vi "test_SimulatedScope SimulatedFGen on MSS ref in parallel.vi"(8 "Error In":errorcluster) -> (0 "Error Out":errorcluster)   [LabVIEW 2023]
uses:
  Measure and Stimulus Subsystems/Measure and Stimulus Subsystems.lvclass
panel:
  out "Photosensor Waveform Chart":waveform(dbl)(graph)
  in  "Stop":bool
  out "Powersensor Scalar":dbl
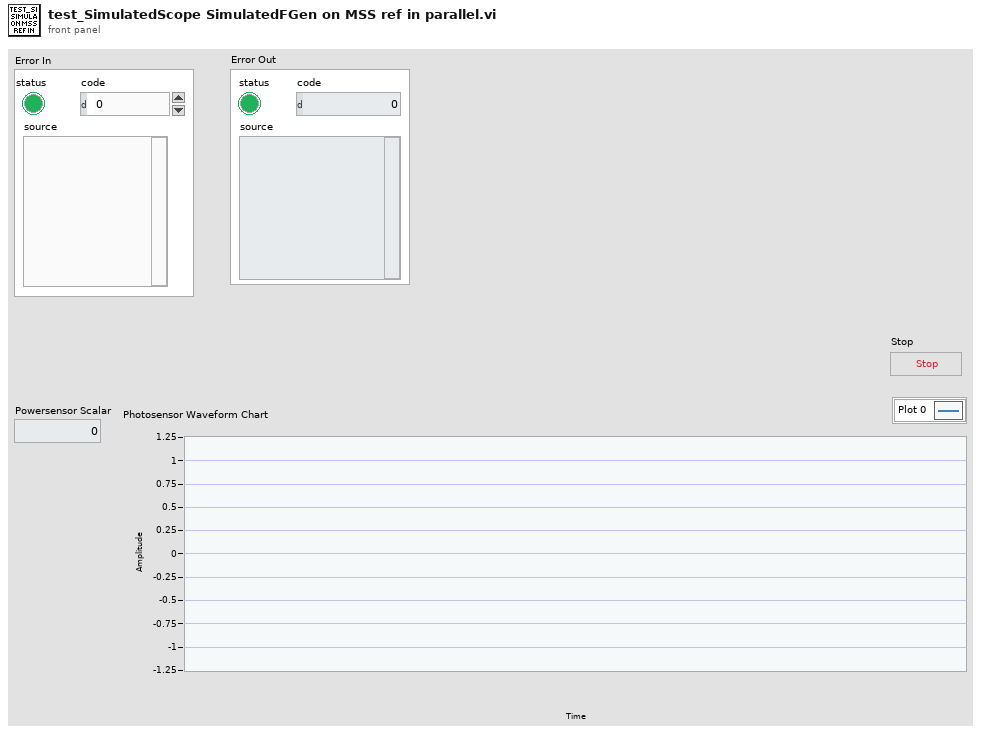
[diagram p1: front panel]
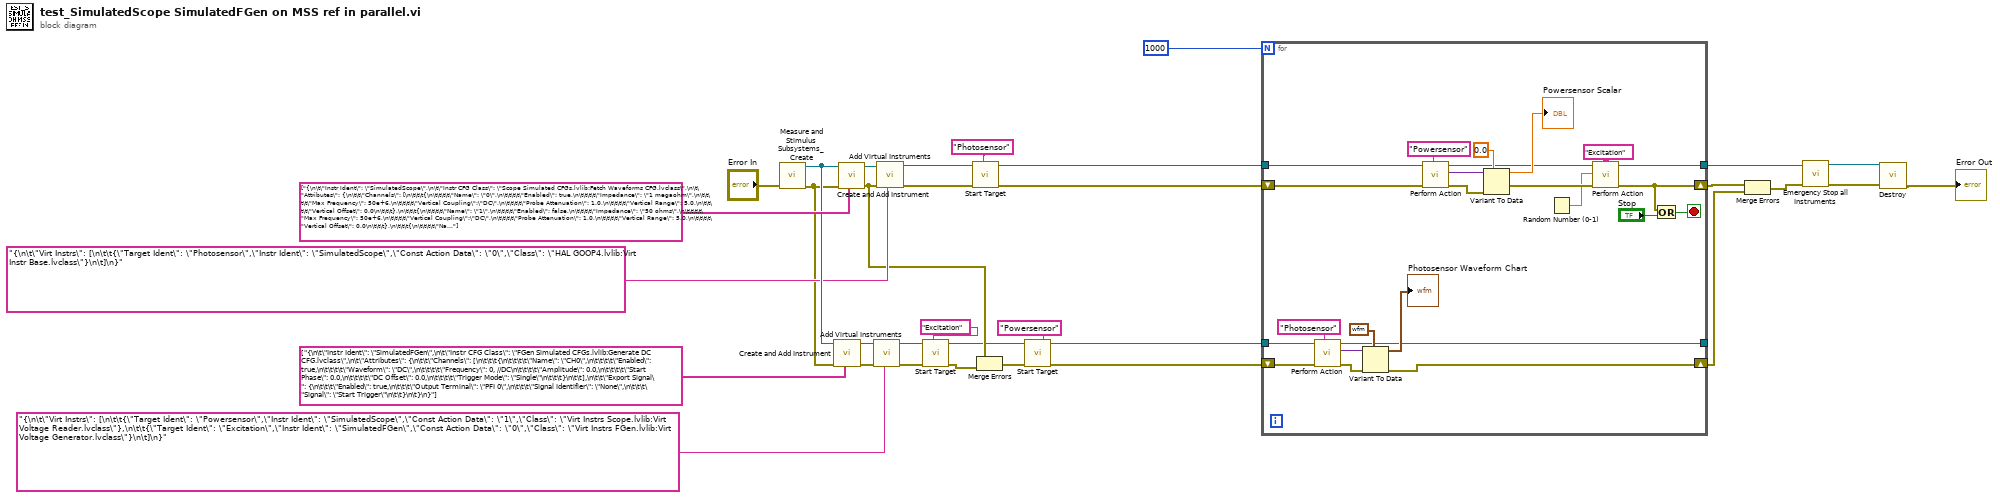
[diagram p0: block diagram]
diagram:
  n1 = call "Measure and Stimulus Subsystems_Create.vi"("Error In"="Error In") -> ("Error Out"=w16:errorcluster, "reference out"=w22:refnum<class "Measure and Stimulus Subsystems.lvclass">)  [unwired: 9 in]
  n2 = call "Create and Add Instrument.vi"("Physical Intr Configs"=string[] ["{\n\t\"Instr Ident\": \"SimulatedFGen\",\n\t\"Instr CFG Class\": \"FGen Simulated CFGs.lvlib:Generate DC CFG.lvclass\",\n\t\"Attributes\": {\n\t\t\"Channels\": [\n\t\t\t{\n\t\t\t\t\"Name\": \"CH0\",\n\t\t\t\t\"Enabled\": true,\n\t\t\t\t\"Waveform\": \"DC\",\n\t\t\t\t\"Frequency\": 0, //DC\n\t\t\t\t\"Amplitude\": 0.0,\n\t\t\t\t\"Start Phase\": 0.0,\n\t\t\t\t\"DC Offset\": 0.0,\n\t\t\t\t\"Trigger Mode\": \"Single\"\n\t\t\t}\n\t\t],\n\t\t\"Export Signal\": {\n\t\t\t\"Enabled\": true,\n\t\t\t\"Output Terminal\": \"PFI 0\",\n\t\t\t\"Signal Identifier\": \"None\",\n\t\t\t\"Signal\": \"Start Trigger\"\n\t\t}\n\t}\n}"], "Error In"=w16, "reference in"=w22) -> ("Error Out"=w15:errorcluster, "reference out"=w14:refnum<class "Measure and Stimulus Subsystems.lvclass">)  [unwired: 7 in]
  n3 = call "Create and Add Instrument.vi"("Physical Intr Configs"=string[] ["{\n\t\"Instr Ident\": \"SimulatedScope\",\n\t\"Instr CFG Class\": \"Scope Simulated CFGs.lvlib:Fetch Waveforms CFG.lvclass\",\n\t\"Attributes\": {\n\t\t\"Channels\": [\n\t\t\t{\n\t\t\t\t\"Name\": \"0\",\n\t\t\t\t\"Enabled\": true,\n\t\t\t\t\"Impedance\": \"1 megaohm\",\n\t\t\t\t\"Max Frequency\": 50e+6,\n\t\t\t\t\"Vertical Coupling\":\"DC\",\n\t\t\t\t\"Probe Attenuation\": 1.0,\n\t\t\t\t\"Vertical Range\": 5.0,\n\t\t\t\t\"Vertical Offset\": 0.0\n\t\t\t},\n\t\t\t{\n\t\t\t\t\"Name\": \"1\",\n\t\t\t\t\"Enabled\": false,\n\t\t\t\t\"Impedance\": \"50 ohms\",\n\t\t\t\t\"Max Frequency\": 50e+6,\n\t\t\t\t\"Vertical Coupling\":\"DC\",\n\t\t\t\t\"Probe Attenuation\": 1.0,\n\t\t\t\t\"Vertical Range\": 5.0,\n\t\t\t\t\"Vertical Offset\": 0.0\n\t\t\t},\n\t\t\t{\n\t\t\t\t\"Name\": \"2\",\n\t\t\t\t\"Enabled\": false,\n\t\t\t\t\"Impedance\": \"50 ohms\",\n\t\t\t\t\"Max Frequency\": 50e+6,\n\t\t\t\t\"Vertical Coupling\":\"DC\",\n\t\t\t\t\"Probe Attenuation\": 1.0,\n\t\t\t\t\"Vertical Range\": 5.0,\n\t\t\t\t\"Vertical Offset\": 0.0\n\t\t\t},\n\t\t\t{\n\t\t\t\t\"Name\": \"3\",\n\t\t\t\t\"Enabled\": true,\n\t\t\t\t\"Impedance\": \"50 ohms\",\n\t\t\t\t\"Max Frequency\": 50e+6,\n\t\t\t\t\"Vertical Coupling\":\"DC\",\n\t\t\t\t\"Probe Attenuation\": 1.0,\n\t\t\t\t\"Vertical Range\": 1.4,\n\t\t\t\t\"Vertical Offset\": 0.0\n\t\t\t},\n\t\t\t{\n\t\t\t\t\"Name\": \"4\",\n\t\t\t\t\"Enabled\": false,\n\t\t\t\t\"Impedance\": \"50 ohms\",\n\t\t\t\t\"Max Frequency\": 50e+6,\n\t\t\t\t\"Vertical Coupling\":\"DC\",\n\t\t\t\t\"Probe Attenuation\": 1.0,\n\t\t\t\t\"Vertical Range\": 5.0,\n\t\t\t\t\"Vertical Offset\": 0.0\n\t\t\t},\n\t\t\t{\n\t\t\t\t\"Name\": \"5\",\n\t\t\t\t\"Enabled\": false,\n\t\t\t\t\"Impedance\": \"50 ohms\",\n\t\t\t\t\"Max Frequency\": 50e+6,\n\t\t\t\t\"Vertical Coupling\":\"DC\",\n\t\t\t\t\"Probe Attenuation\": 1.0,\n\t\t\t\t\"Vertical Range\": 5.0,\n\t\t\t\t\"Vertical Offset\": 0.0\n\t\t\t},\n\t\t\t{\n\t\t\t\t\"Name\": \"6\",\n\t\t\t\t\"Enabled\": false,\n\t\t\t\t\"Impedance\": \"50 ohms\",\n\t\t\t\t\"Max Frequency\": 50e+6,\n\t\t\t\t\"Vertical Coupling\":\"DC\",\n\t\t\t\t\"Probe Attenuation\": 1.0,\n\t\t\t\t\"Vertical Range\": 5.0,\n\t\t\t\t\"Vertical Offset\": 0.0\n\t\t\t},\n\t\t\t{\n\t\t\t\t\"Name\": \"7\",\n\t\t\t\t\"Enabled\": false,\n\t\t\t\t\"Impedance\": \"50 ohms\",\n\t\t\t\t\"Max Frequency\": 50e+6,\n\t\t\t\t\"Vertical Coupling\":\"DC\",\n\t\t\t\t\"Probe Attenuation\": 1.0,\n\t\t\t\t\"Vertical Range\": 5.0,\n\t\t\t\t\"Vertical Offset\": 0.0\n\t\t\t}\n\t\t],\n\t\t\"Horizontal\": {\n\t\t\t\"Enforce Realtime\": true,\n\t\t\t\"Number of Records\": 1,\n\t\t\t\"Min Sample Rate\": 1e+5,\n\t\t\t\"Reference Position\":50, //percent\n\t\t\t\"Min Record Length\":1e+3\n\t\t},\n\t\t\"Acquire\": {\n\t\t\t\"Type\": \"Normal\",\n\t\t\t\"NumSamples\": 1e+3,\n\t\t\t\"Fetch Relative To\": \"Read Pointer\"\n\t\t},\n\t\t\"Export Signal\": {\n\t\t\t\"Signal Identifier\": \"None\",\n\t\t\t\"Signal\": \"None\",\n\t\t\t\"Output Terminal\": \"None\"\n\t\t},\n\t\t\"Trigger\": {\n\t\t\t\"Type\": \"Immediate\",\n\t\t\t\"Slope\": \"Positive\",\n\t\t\t\"Source\": \"RTSI 0\",\n\t\t\t\"Holdoff\": 0.0,\n\t\t\t\"Delay\": 0.0\n\t\t}\n\t}\n}"], "Error In"=w16, "reference in"=w22) -> ("Error Out"=w7:errorcluster, "reference out"=w20:refnum<class "Measure and Stimulus Subsystems.lvclass">)  [unwired: 7 in]
  n4 = call "Add Virtual Instruments.vi"("<JSON CFG>"="{\n\t\"Virt Instrs\": [\n\t\t{\"Target Ident\": \"Powersensor\",\"Instr Ident\": \"SimulatedScope\",\"Const Action Data\": \"1\",\"Class\": \"Virt Instrs Scope.lvlib:Virt Voltage Reader.lvclass\"},\n\t\t{\"Target Ident\": \"Excitation\",\"Instr Ident\": \"SimulatedFGen\",\"Const Action Data\": \"0\",\"Class\": \"Virt Instrs FGen.lvlib:Virt Voltage Generator.lvclass\"}\n\t]\n}", "Error In"=w15, "reference in"=w14) -> ("Error Out"=w9:errorcluster, "reference out"=w10:refnum<class "Measure and Stimulus Subsystems.lvclass">)  [unwired: 7 in]
  n5 = call "Add Virtual Instruments.vi"("<JSON CFG>"="{\n\t\"Virt Instrs\": [\n\t\t{\"Target Ident\": \"Photosensor\",\"Instr Ident\": \"SimulatedScope\",\"Const Action Data\": \"0\",\"Class\": \"HAL GOOP4.lvlib:Virt Instr Base.lvclass\"}\n\t]\n}", "Error In"=w7, "reference in"=w20) -> ("Error Out"=w21:errorcluster, "reference out"=w19:refnum<class "Measure and Stimulus Subsystems.lvclass">)  [unwired: 7 in]
  n6 = call "Start Target.vi"("Target Ident"="Excitation", "Error In"=w9, "reference in"=w10) -> ("Error Out"=w6:errorcluster, "reference out"=w5:refnum<class "Measure and Stimulus Subsystems.lvclass">)  [unwired: 7 in]
  n7 = call "Start Target.vi"("Target Ident"="Photosensor" ("Target Identifier"), "Error In"=w21, "reference in"=w19) -> ("Error Out"=w12:errorcluster, "reference out"=w25:refnum<class "Measure and Stimulus Subsystems.lvclass">)  [unwired: 7 in]
  n8 = Merge Errors(w7, w6) -> (w8:errorcluster)
  n9 = call "Start Target.vi"("Target Ident"="Powersensor" ("Target Identifier"), "Error In"=w8, "reference in"=w5) -> ("Error Out"=w3:errorcluster, "reference out"=w4:refnum<class "Measure and Stimulus Subsystems.lvclass">)  [unwired: 7 in]
  n10 = for {
    N: 1000 -> [_]
    shift-right: [w47] -> w29
    shift-left: w12 -> [w55]
    tunnel: w4 -> [w37]
    shift-right: [w35] -> w1
    shift-left: w3 -> [w36]
    tunnel: [w34] -> _
    tunnel: w25 -> [w54]
    tunnel: [w45] -> w32
    stop <- w48 stop-if-true
    n11 = call "Perform Action.vi"("Target Ident"="Photosensor" ("Target Identifier"), "Error In"=w36, "reference in"=w37) -> ("Error Out"=w39:errorcluster, "Output"=w40:variant, "reference out"=w34:refnum<class "Measure and Stimulus Subsystems.lvclass">)  [unwired: 6 in]
    n12 = Variant To Data(error in=w39, type=waveform(dbl) {"t0"=timestamp(0 s since 1904-01-01), "dt"=1.0, "Y"=[]} ("Waveform"), Variant=w40) -> (data=→"Photosensor Waveform Chart":waveform(dbl), error out=w35:errorcluster)
    n13 = call "Perform Action.vi"("Target Ident"="Powersensor" ("Target Identifier"), "Error In"=w55, "reference in"=w54) -> ("Error Out"=w56:errorcluster, "Output"=w53:variant, "reference out"=w46:refnum<class "Measure and Stimulus Subsystems.lvclass">)  [unwired: 6 in]
    n14 = Variant To Data(error in=w56, type=0.0, Variant=w53) -> (data=→"Powersensor Scalar":dbl, error out=w49:errorcluster)
    n15 = Random Number (0-1)() -> (number: 0 to 1=w43:dbl)
    n16 = call "Perform Action.vi"("Target Ident"="Excitation", "Error In"=w49, "Input"=w43, "reference in"=w46) -> ("Error Out"=w47:errorcluster, "reference out"=w45:refnum<class "Measure and Stimulus Subsystems.lvclass">)  [unwired: 5 in, 1 out]
    n17 = Or(x=w47, y="Stop") -> (x .or. y?=w48:bool)
  }
  n18 = Merge Errors(w29, w1) -> (w2:errorcluster)
  n19 = call "Emergency Stop all Instruments.vi"("Error In"=w2, "reference in"=w32) -> ("Error Out"=w33:errorcluster, "reference out"=w31:refnum<class "Measure and Stimulus Subsystems.lvclass">)  [unwired: 8 in]
  n20 = call "Destroy.vi"("Error In"=w33, "reference in"=w31) -> ("Error Out"=→"Error Out":errorcluster)  [unwired: 8 in, 1 out]
